vi "Get Base.vi"(11 "Default Value":string) -> (2 "Number Base":u8, 3 "Default Value (dup)":string)   [LabVIEW 2024, in "EDS.lvlib"]
doc: "Return number base of a string (10 for desimal, 16 for hex and 8 for octal)"
uses:
  EDS.lvlib
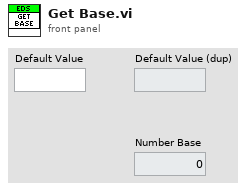
[diagram p1: front panel]
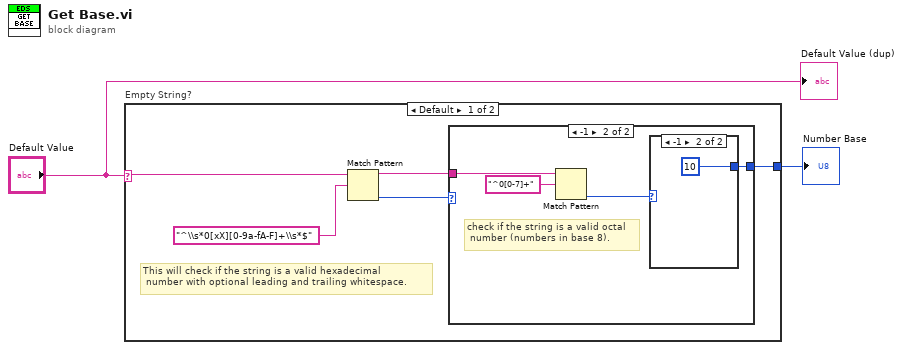
[diagram p0: block diagram]
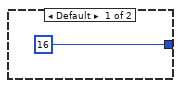
[diagram p2: hidden frame]
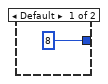
[diagram p3: hidden frame]
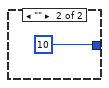
[diagram p4: hidden frame]
diagram:
  n1 = case "Empty String?" shown="Default" "Default Value" {
    selector: "Default Value" -> [w7 _]
    tunnel: [w4 u8 10] -> w2
    frame Default {
      # "This will check if the string is a valid hexadecimal\n number with optional leading and trailing whitespace."
      n2 = Match Pattern(string=w7, regular expression="^\\s*0[xX][0-9a-fA-F]+\\s*$") -> (before substring=w3:string, offset past match=w5:i32)  [unwired: 1 in, 2 out]
      n3 = case shown="-1" w5 {
        tunnel: [u8 16 w10] -> w4
        tunnel: w3 -> [_ w12]
        frame Default {
        }
        frame -1 {
          # "check if the string is a valid octal\n number (numbers in base 8)."
          n4 = Match Pattern(string=w12, regular expression="^0[0-7]+") -> (offset past match=w9:i32)  [unwired: 1 in, 3 out]
          n5 = case shown="-1" w9 {
            tunnel: [u8 8 u8 10] -> w10
            frame Default {
            }
            frame -1 {
            }
          }
        }
      }
    }
    frame "" {
    }
  }
  "Number Base" <- w2
  "Default Value (dup)" <- "Default Value"
